vi "Set Expires In.vi"(10 "Expires In":dbl, 11 "Authorization in":refnum<class "Authorization.lvclass">) -> (3 "Authorization out":refnum<class "Authorization.lvclass">)   [LabVIEW 2020, in "OAuth2.lvlib" / "Authorization.lvclass"]
doc: "This is an internal VI only necessary when creating new Authorization logic. This is written from the expiry timeout returned by the authorization provider when access was granted."
uses:
  Authorization.lvclass
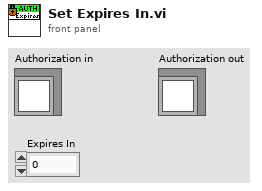
[diagram p1: front panel]
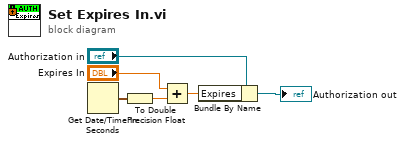
[diagram p0: block diagram]
diagram:
  n1 = Get Date/Time In Seconds() -> (seconds since 1Jan1904=w5:timestamp)
  n2 = To Double Precision Float(number=w5) -> (double precision float=w3:dbl)
  n3 = Add(x="Expires In", y=w3) -> (x+y=w1:dbl)
  n4 = Bundle By Name(cluster="Authorization in", "Expires"=w1) -> (→"Authorization out":refnum<class "Authorization.lvclass">)
